vi "Cycle Images.vi"(0 "Image Path":path=path "C:/Users/serce/Desktop/Smart Vision System Testbench/Test Images/P3_Side0000.png", 4 "Number of Images":i32=12, 7 "error in":errorcluster) -> (20 "Image Out":T1(plugin-control), 21 "All Images Out":T1[](array[typedef]), 26 "Stopped":bool, 27 "error out":errorcluster)   [LabVIEW 2020]
doc: "Creates, and edits acquisitions using the NI Vision Acquisition Express VI.\n\nThe NI Vision Acquisition Wizard is launched by placing the Express VI on the block diagram. Select an acquisition source and configure an acquisition using NI-IMAQ, NI-IMAQdx, or simulate an acquisition by reading an AVI or image files from a folder. After an acquisition is configured, select controls and indicators to be able to programmatically set in LabVIEW. Double-click the Vision Acquisition Express VI to edit the acquisition.\n\nNote: Any images created by the Express VI need to be disposed after use. Use the IMAQ Dispose.vi to cleanup the images output by the Express VI when they are no longer needed."
uses:
  <vilib>/vision/Image Controls.llb/IMAQ Image.ctl
  <vilib>/vision/driver/Vision Acquisition Express Utility VIs.llb/Vision Acquisition Path Convert (Path).vi
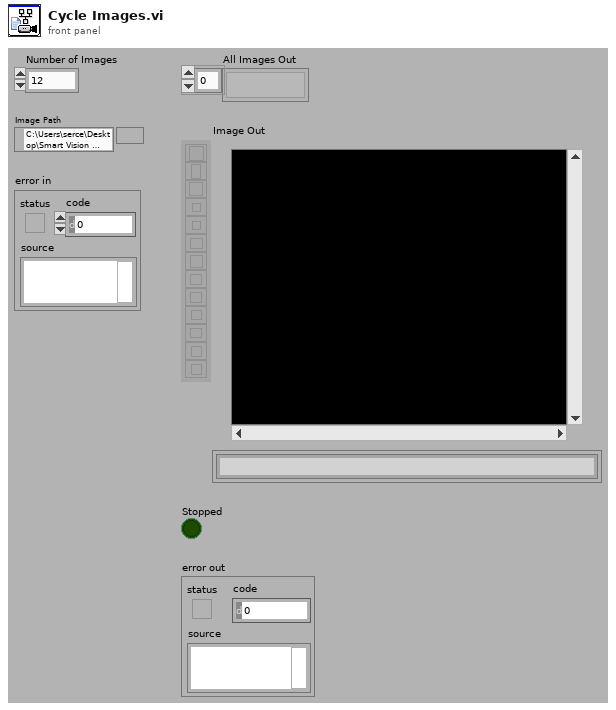
[diagram p1: front panel]
types:
  T1 = typedef "IMAQ Image.ctl" = refnum<image>
  T2 = typedef "Image Type" = u32
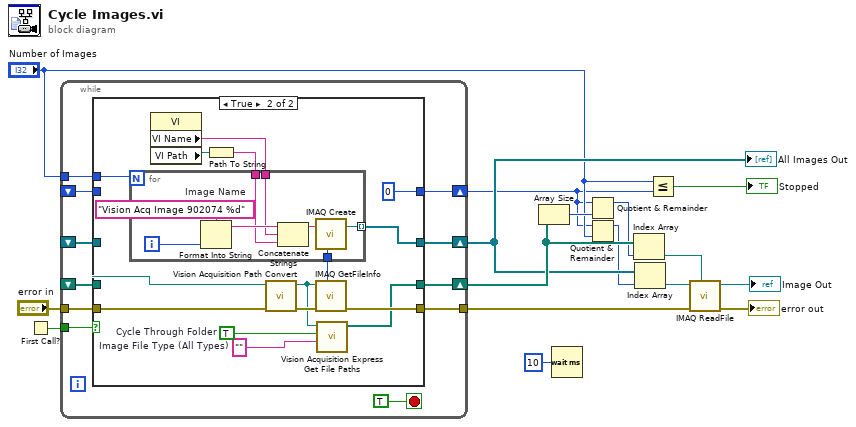
[diagram p0: block diagram]
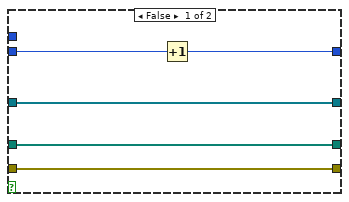
[diagram p2: hidden frame]
diagram:
  n1 = First Call?() -> (First Call?: T/F=w16:bool)
  n2 = while "While Loop_template0_template0" {
    shift-right: [w26] -> w12
    shift-left: _ -> [w25]
    tunnel: w16 -> [w27]
    tunnel: [w24] -> w13
    tunnel: "error in" -> [w23]
    shift-right: [w21] -> w8
    shift-left: _ -> [w20]
    tunnel: "Number of Images" -> [w19]
    shift-right: [w18] -> w2
    shift-left: _ -> [w17]
    stop <- TRUE ("_template0_template0") stop-if-true
    n3 = case "Case Structure_template0_template0" shown="True" w27 {
      tunnel: [w32 w40] -> w26
      tunnel: w25 -> [w32 _]
      tunnel: [w31 w45] -> w24
      tunnel: w23 -> [w31 w44]
      tunnel: [w30 w46] -> w21
      tunnel: w20 -> [w30 _]
      tunnel: w19 -> [_ w43]
      tunnel: [w28 0] -> w18
      tunnel: w17 -> [w29 _]
      frame False {
        n4 = Increment(x=w29) -> (x+1=w28:i32)
      }
      frame True {
        w35 = ""  # Image File Type (All Types)
        w41 = TRUE  # Cycle Through Folder
        n5 = property class="VI"() -> ("VI Name"=w37:string, "VI Path"=w38:path)  [unwired: 2 in, 2 out]
        n6 = Path To String(path=w38) -> (string=w36:string)
        n7 = call-poly <vilib>:"Vision Acquisition Path Convert.vi"("Path In"="Image Path") -> ("Path Out"=w34:path)  [unwired: 10 in]
        n8 = call "IMAQ GetFileInfo"("error in (no error)"=w44, "File Path"=w34) -> ("error out"=w45:errorcluster, "Image Type"=w42:T2)  [unwired: 8 out]
        n9 = for {
          N: w43 -> [_]
          tunnel: w42 -> [w54]
          tunnel: [w53] -> w46 mode=indexing
          tunnel: w37 -> [w49]
          tunnel: w36 -> [w47]
          i -> [w52]
          w51 = "Vision Acq Image 902074 %d"  # Image Name
          n10 = Format Into String(format string=w51, w52) -> (resulting string=w50:string)  [unwired: 2 in, 1 out]
          n11 = Concatenate Strings(w50, w49, w47) -> (w48:string)
          n12 = call "IMAQ Create"("Image Name"=w48, "Image Type"=w54) -> ("New Image"=w53:T1)  [unwired: 2 in, 2 out]
        }
        n13 = call <vilib>:"Vision Acquisition Express Get File Paths.vi"("Image File Type (All Types)"=w35, "Cycle Through Folder"=w41, "File Path"=w34) -> ("File Paths"=w40:path[])  [unwired: 8 out]
      }
    }
  }
  "All Images Out" <- w8
  n14 = Array Size(array=w12) -> (size(s)=w14:i32)
  n15 = Wait (ms)(milliseconds to wait=u32 10) -> ()  [unwired: 1 out]
  n16 = Quotient & Remainder(x=w2, y=w14) -> (x-y*floor(x/y)=w11:i32)  [unwired: 1 out]
  n17 = Quotient & Remainder(x=w2, y="Number of Images") -> (x-y*floor(x/y)=w7:i32)  [unwired: 1 out]
  n18 = Index Array(array=w12, index=w11) -> (element=w10:path)
  n19 = Index Array(array=w8, index=w7) -> (element=w6:T1)
  n20 = Less Or Equal?(x="Number of Images", y=w2) -> (x <= y?=→"Stopped":bool)
  n21 = call "IMAQ ReadFile"("File Path"=w10, "error in (no error)"=w13, "Image"=w6) -> ("error out"=→"error out":errorcluster, "Image Out"=→"Image Out":T1)  [unwired: 2 in, 5 out]
